vi "Acnet Device Writer RPC.vi"(1 "Value":string="192.7", 2 "Device":string="D:BPJ10D") -> ()   [LabVIEW 2013]
panel:
  out "error out":errorcluster
  out "String length":i32=221
  in  "Preamble":string="POST /xmlrpc/Accelerator HTTP/1.0\r\nContent-Type: text/xml\r\nContent-Length: "
  in  "remote port":u16=4352
  in  "Data in 3":string="</double></value>\n</param>\n\n</params>\n</methodCall>"
  in  "Data in 2":string="</string></value>\n</param>\n<param>\n<value><double>"
  in  "address":string="dce34.fnal.gov"
  out "data out":string="HTTP/1.0 200 OK\r\nServer: Apache XML-RPC 1.0\r\nConnection: close\r\nContent-Type: text/xml\r\nContent-Length: 135\r\n\r\n<?xml version=\"1.0\" encoding=\"ISO-8859-1\"?><methodResponse><params><param><value><int>0</int></value></param></params></methodResponse>"
  in  "Data in":string="<?xml version='1.0'?>\n<methodCall>\n<methodName>Remote.setting</methodName>\n<params>\n<param>\n<value><string>"
  # "Acnet Device Writer\nupdated 5 Mar 2013\nby D. Peterson"
  # "2/23/06\nWrites value to Acnet device via DUE."
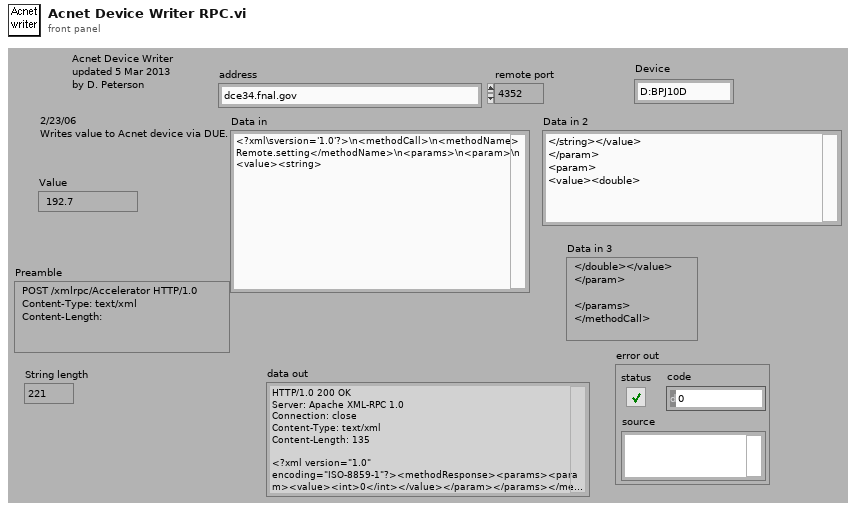
[diagram p1: front panel]
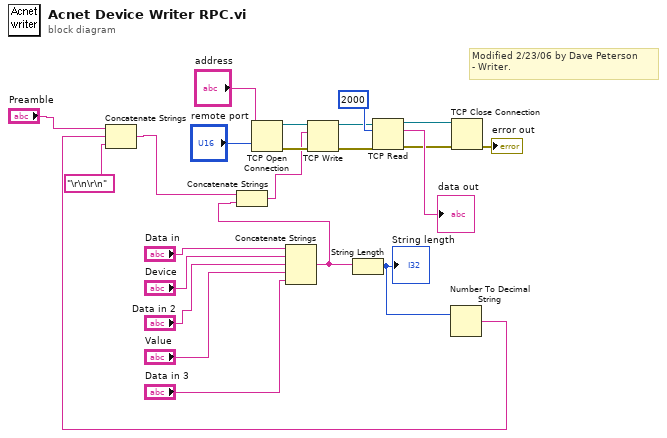
[diagram p0: block diagram]
diagram:
  # "Modified 2/23/06 by Dave Peterson\n- Writer."
  n1 = TCP Open Connection(address="address", remote port or service name="remote port") -> (connection ID=w23:refnum<k5>, error out=w22:errorcluster)  [unwired: 3 in]
  n2 = Concatenate Strings("Data in", "Device", "Data in 2", "Value", "Data in 3") -> (w5:string)
  n3 = String Length(string=w5) -> (length=w4:i32)
  "String length" <- w4
  n4 = Number To Decimal String(number=w4) -> (decimal integer string=w2:string)  [unwired: 1 in]
  n5 = Concatenate Strings("Preamble", w2, "\r\n\r\n" ("string")) -> (w6:string)
  n6 = Concatenate Strings(w6, w5) -> (w7:string)
  n7 = TCP Write(connection ID=w23, data in=w7, error in (no error)=w22) -> (connection ID out=w19:refnum<k5>, error out=w18:errorcluster)  [unwired: 1 in, 1 out]
  n8 = TCP Read(connection ID=w19, bytes to read=2000, error in (no error)=w18) -> (connection ID out=w12:refnum<k5>, data out=→"data out":string, error out=w13:errorcluster)  [unwired: 2 in]
  n9 = TCP Close Connection(connection ID=w12, error in (no error)=w13) -> (error out=→"error out":errorcluster)  [unwired: 1 in, 1 out]
